vi "Get Routing Channel by Name.vi"(8 "error in (no error)":errorcluster, 10 "Channel Name":string, 11 "Routing Channels Ref in":T1 format="%.0x") -> (0 "error out":errorcluster, 2 "Channel Ref":T1 format="%.0x", 3 "Routing Channels Ref out":T1 format="%.0x")   [LabVIEW 2017, in "Routing and Faulting Scripting.lvlib"]
uses:
  Routing and Faulting Scripting.lvlib
  <vilib>/NI Veristand/Custom Device API/Custom Device Item Ref.ctl
  <vilib>/NI VeriStand/Custom Device API/Custom Device API.lvlib
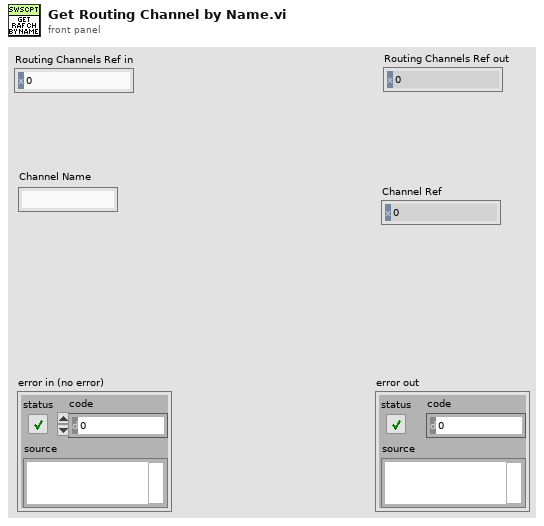
[diagram p1: front panel]
types:
  T1 = typedef "Custom Device API.lvlib/Custom Device Item Ref.ctl" = u64
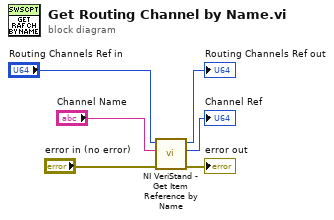
[diagram p0: block diagram]
diagram:
  n1 = call <vilib>:"NI VeriStand - Get Item Reference by Name.vi"("error in (no error)"="error in (no error)", "Item Name"="Channel Name", "Parent Ref in"="Routing Channels Ref in") -> ("error out"=→"error out":errorcluster, "Item Ref"=→"Channel Ref":T1, "Parent Ref out"=→"Routing Channels Ref out":T1)  [unwired: 5 in, 1 out]
